vi "Untitled 1.vi"   [LabVIEW 2019]
types:
  T1 = enum16{"open", "replace", "create", "open or create", "replace or create", "replace or create with confirmation"}
  T2 = typedef "Eth timeouts.ctl" = cluster{"conn_timeout":i32, "reconn_timeout":i32, "N attempt max":i32, "t_reset_TTL":i32, "write_timeout":i32, "read_timeout":i32, "period":i32}
  T3 = cluster{"Remote IP Address":string, "Remote Port":u16}[]
  T4 = cluster{"MVIName def":string[], "IP addr def":cluster{"Remote IP Address":string, "Remote Port":u16}[], "timeouts def":T2[], "start_stop def":bool[], "WR en def":bool[]}
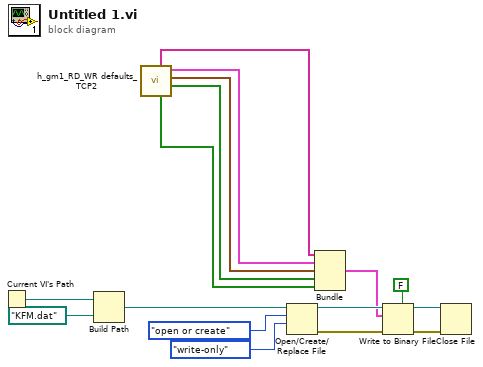
[diagram p0: block diagram]
diagram:
  n1 = Current VI's Path() -> (path=w13:path)
  n2 = Build Path(base path=w13, name or relative path=path "KFM.dat" ("file (use dialog)")) -> (appended path=w12:path)
  n3 = call "h_gm1_RD_WR defaults_TCP2.vi"() -> ("start_stop def"=w8:bool[], "timeouts def"=w9:T2[], "IP addr def"=w10:T3, "WR en def"=w7:bool[], "MVIName def"=w1:string[])  [unwired: 7 in]
  n4 = Open/Create/Replace File(file path (use dialog)=w12, operation (0:open)=T1."open or create", access (0:read/write)=enum16{"read/write", "read-only", "write-only"}."write-only") -> (refnum out=w11:refnum<file>, error out=w4:errorcluster)  [unwired: 3 in, 1 out]
  n5 = Bundle("MVIName def"=w1, "IP addr def"=w10, "timeouts def"=w9, "start_stop def"=w8, "WR en def"=w7) -> (w5:T4)  [unwired: 1 in]
  n6 = Write to Binary File(file (use dialog)=w11, data=w5, error in=w4, 5:FALSE ("prepend array or string size? (T)")) -> (refnum out=w3:refnum<file>, error out=w2:errorcluster)  [unwired: 2 in, 1 out]
  n7 = Close File(refnum=w3, error in=w2) -> ()  [unwired: 2 out]
